vi "hpanel_delete_user_events.vi"(8 "error in (no error)":errorcluster, 11 "hydraharp_panel in":refnum<class "hydraharp_panel.lvclass">) -> (0 "error out":errorcluster, 3 "hydraharp_panel out":refnum<class "hydraharp_panel.lvclass">)   [LabVIEW 2015, in "hydraharp_panel.lvclass"]
uses:
  hydraharp_panel.lvclass
  hydraharp_panel.lvclass/hydraharp_panel.ctl
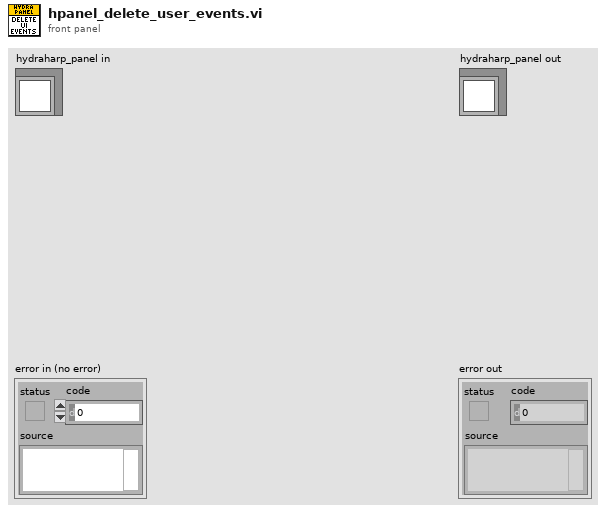
[diagram p1: front panel]
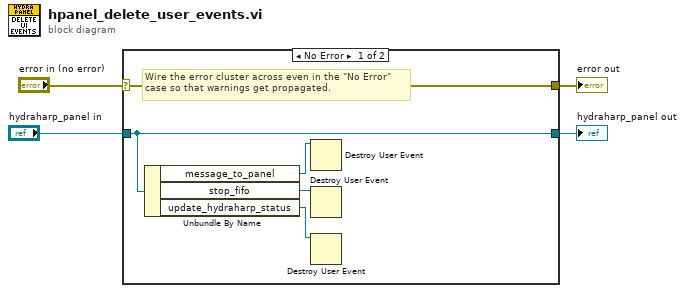
[diagram p0: block diagram]
diagram:
  n1 = case shown="No Error" "error in (no error)" {
    selector: "error in (no error)" -> [w9 w11]
    tunnel: [w9 w11] -> w3
    tunnel: [w8 w10] -> w1
    tunnel: "hydraharp_panel in" -> [w8 w10]
    frame No Error {
      # "Wire the error cluster across even in the \"No Error\"\ncase so that warnings get propagated."
      n2 = Unbundle By Name(w8) -> ("message_to_panel"=w7:refnum<user-event>, "stop_fifo"=w6:refnum<user-event>, "update_hydraharp_status"=w5:refnum<user-event>)
      n3 = Destroy User Event(user event=w7) -> ()  [unwired: 1 in, 1 out]
      n4 = Destroy User Event(user event=w6) -> ()  [unwired: 1 in, 1 out]
      n5 = Destroy User Event(user event=w5) -> ()  [unwired: 1 in, 1 out]
    }
    frame Error {
    }
  }
  "error out" <- w3
  "hydraharp_panel out" <- w1
